vi "-8334 Table display name must begin with either a letter or underscore or backlash--error.vi"(8 "error in":errorcluster, 11 "Argument":string) -> (0 "error out":errorcluster, 2 "Error Code":i32)   [LabVIEW 2019, in "Open Xml.lvlib"]
uses:
  Open Xml.lvlib
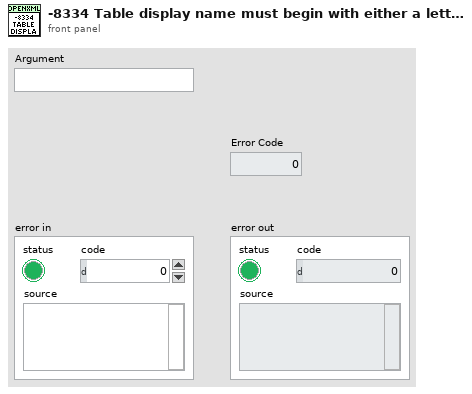
[diagram p1: front panel]
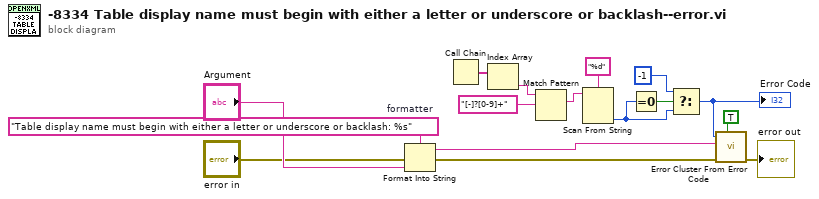
[diagram p0: block diagram]
diagram:
  w13 = "Table display name must begin with either a letter or underscore or backlash: %s"  # formatter
  n1 = Format Into String(format string=w13, error in="error in", "Argument") -> (resulting string=w14:string, error out=w2:errorcluster)  [unwired: 1 in]
  n2 = Call Chain() -> (call chain=w4:string[])
  n3 = Index Array(array=w4) -> (element=w9:string)  [unwired: 1 in]
  n4 = Match Pattern(string=w9, regular expression="[-]?[0-9]+") -> (match substring=w10:string)  [unwired: 1 in, 3 out]
  n5 = Scan From String(format string="%d", input string=w10) -> (output 1=w6:i32)  [unwired: 3 in, 3 out]
  n6 = Equal To 0?(x=w6) -> (x = 0?=w7:bool)
  n7 = Select(t=-1, s=w7, f=w6) -> (s? t:f=w1:i32)
  "Error Code" <- w1
  n8 = call <vilib>:"Error Cluster From Error Code.vi"("show call chain? (False)"=TRUE, "error in (no error)"=w2, "error message (\"\")"=w14, "error code (0)"=w1) -> ("error out"=→"error out":errorcluster)  [unwired: 5 in]
